vi "cameraclose.vi"   [LabVIEW 2026]
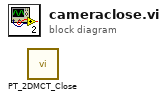
[diagram p0: block diagram]
diagram:
  n1 = call "PT_2DMCT_Close.vi"() -> ()  [unwired: 11 in, 1 out]
